vi "SpdCmdGenerate.vi"(1 "Speed":sgl=1.5 format="%.4f") -> (0 "CMD code":string)   [LabVIEW 2012]
panel:
  out "Revised":u8[](array[numeric]) format="%02x"
  out "Array":u8[](array[numeric]) format="%02x"
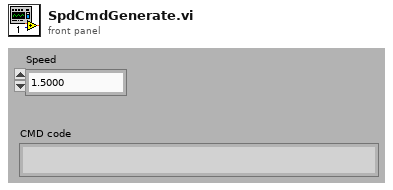
[diagram p1: front panel]
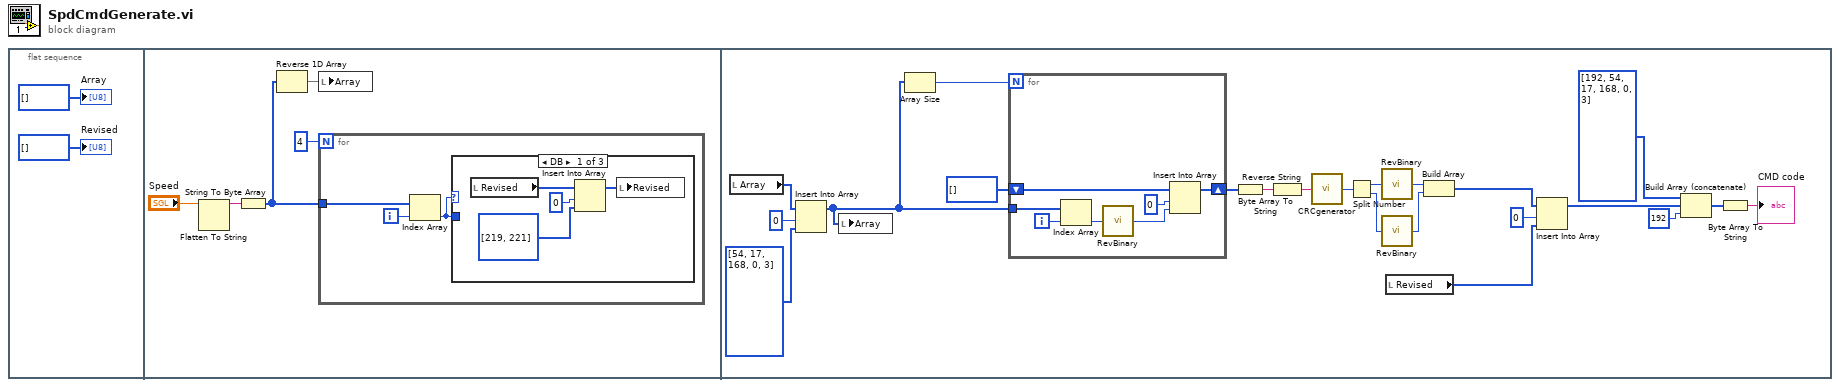
[diagram p0: block diagram]
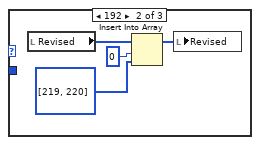
[diagram p2: hidden frame]
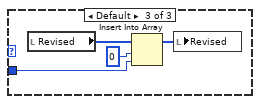
[diagram p3: hidden frame]
diagram:
  n1 = flat-sequence {
    frame #0 {
      "Array" <- u8[] []
      "Revised" <- u8[] []
    }
    frame #1 {
      n2 = Flatten To String(anything="Speed") -> (data string=w6:string)  [unwired: 3 in, 2 out]
      n3 = String To Byte Array(string=w6) -> (unsigned byte array=w4:u8[])
      n4 = Reverse 1D Array(array=w4) -> (reversed array=w3:u8[])
      n5 = local write "Array"(w3) -> ()
      n6 = for {
        N: 4 -> [_]
        tunnel: w4 -> [w9]
        i -> [w10]
        n7 = Index Array(array=w9, index=w10) -> (element=w8:u8)
        n8 = case shown="DB" w8 {
          tunnel: w8 -> [_ _ w22]
          frame 219 {
            n9 = local read "Revised"() -> (w11:u8[])
            n10 = Insert Into Array(array=w11, index=0, new element=i32[] [219, 221]) -> (w13:u8[])
            n11 = local write "Revised"(w13) -> ()
          }
          frame 192 {
            n12 = local read "Revised"() -> (w16:u8[])
            n13 = Insert Into Array(array=w16, index=0, new element=i32[] [219, 220]) -> (w15:u8[])
            n14 = local write "Revised"(w15) -> ()
          }
          frame Default {
            n15 = local read "Revised"() -> (w19:u8[])
            n16 = Insert Into Array(array=w19, index=0, new element=w22) -> (w21:u8[])
            n17 = local write "Revised"(w21) -> ()
          }
        }
      }
    }
    frame #2 {
      n18 = local read "Array"() -> (w44:u8[])
      n19 = Insert Into Array(array=w44, index=0, new element=i32[] [54, 17, 168, 0, 3]) -> (w40:u8[])
      n20 = local write "Array"(w40) -> ()
      n21 = Array Size(array=w40) -> (size(s)=w41:i32)
      n22 = for {
        N: w41 -> [_]
        tunnel: w40 -> [w51]
        shift-right: [w48] -> w36
        shift-left: u32[] [] -> [w47]
        i -> [w50]
        n23 = Index Array(array=w51, index=w50) -> (element=w46:u8)
        n24 = call "RevBinary.vi"("Binary"=w46) -> ("Rev Binary"=w45:u32)
        n25 = Insert Into Array(array=w47, index=0, new element=w45) -> (w48:u32[])
      }
      n26 = Byte Array To String(unsigned byte array=w36) -> (string=w37:string)
      n27 = Reverse String(1:w37) -> (0:w38:string)
      n28 = call "CRCgenerator.vi"("String"=w38) -> ("CRC-16-CCITT-0xFFFF"=w35:u16)
      n29 = Split Number(x=w35) -> (hi(x)=w34:u8, lo(x)=w33:u8)
      n30 = call "RevBinary.vi"("Binary"=w34) -> ("Rev Binary"=w30:u32)
      n31 = call "RevBinary.vi"("Binary"=w33) -> ("Rev Binary"=w29:u32)
      n32 = local read "Revised"() -> (w31:u8[])
      n33 = Build Array(w30, w29) -> (w28:u32[])
      n34 = Insert Into Array(array=w28, index=0, new element=w31) -> (w24:u32[])
      n35 = Build Array (concatenate)(i32[] [192, 54, 17, 168, 0, 3], w24, 192) -> (w27:u32[])
      n36 = Byte Array To String(unsigned byte array=w27) -> (string=→"CMD code":string)
    }
  }
